vi "Pix Diff and Angle Info.vi"(6 "Split Image Info":T3={"height"=120.0, "width"=120.0, "deg/pix"=120.0}, 10 "Angle Mode":enum16{"Barrel View", "360 View"}(ring), 11 "located tags":T2(array[cluster])) -> ()   [LabVIEW 2025]
panel:
  out "angle":dbl
  in  "deg/pix":dbl=0.125
  out "X":dbl
  out "Array 2":cluster{"X":dbl, "Y":dbl}[](array[cluster])
  out "Array":T1(array[cluster])
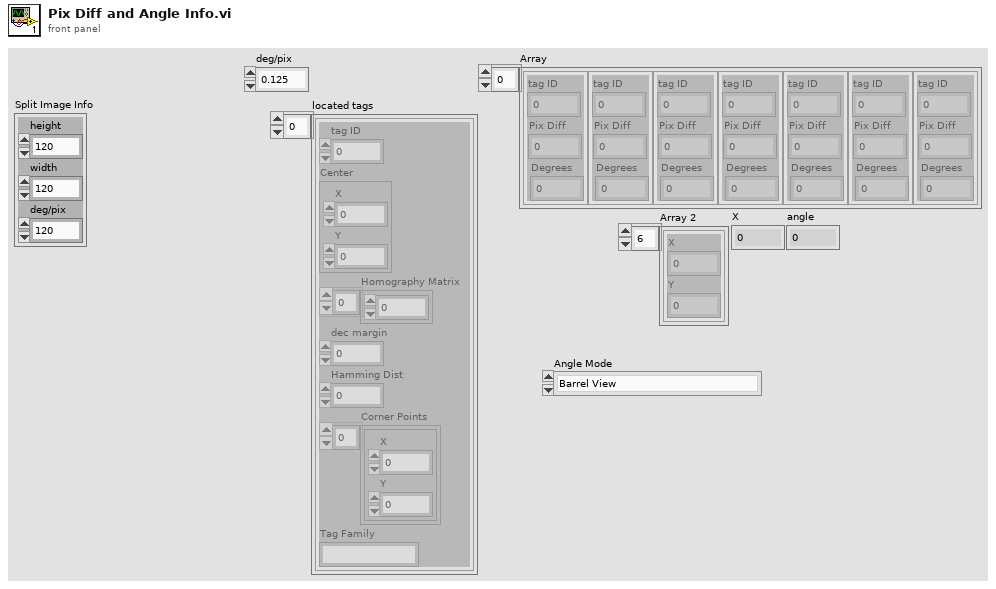
[diagram p1: front panel]
types:
  T1 = cluster{"tag ID":i32, "Pix Diff":dbl, "Degrees":dbl}[]
  T2 = cluster{"tag ID":i32, "Center":cluster{"X":dbl, "Y":dbl}, "Homography Matrix":dbl[], "dec margin":dbl, "Hamming Dist":i32, "Corner Points":cluster{"X":dbl, "Y":dbl}[], "Tag Family":string}[]
  T3 = cluster{"height":dbl, "width":dbl, "deg/pix":dbl}
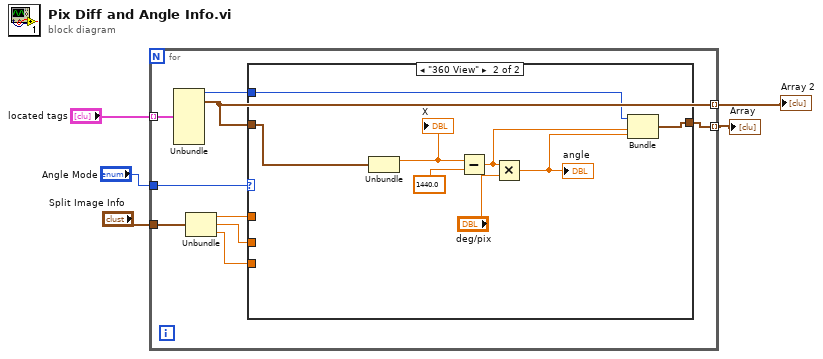
[diagram p0: block diagram]
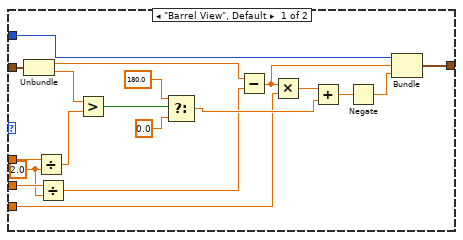
[diagram p2: hidden frame]
diagram:
  n1 = for {
    tunnel: "Split Image Info" -> [w14]
    tunnel: "located tags" -> [w10] mode=indexing
    tunnel: [w9] -> w3 mode=indexing
    tunnel: [w7] -> w2 mode=indexing
    tunnel: "Angle Mode" -> [w6]
    n2 = Unbundle(w10) -> ("tag ID"=w8:i32, "Center"=w7:cluster{"X":dbl, "Y":dbl})  [unwired: 5 out]
    n3 = Unbundle(w14) -> ("height"=w12:dbl, "width"=w13:dbl, "deg/pix"=w11:dbl)
    n4 = case shown="\"360 View\"" w6 {
      tunnel: w13 -> [w25 _]
      tunnel: w12 -> [w24 _]
      tunnel: w11 -> [w20 _]
      tunnel: [w19 w34] -> w9
      tunnel: w8 -> [w16 w37]
      tunnel: w7 -> [w15 w38]
      frame "Barrel View", Default {
        w23 = 2.0 ("y")
        n5 = Unbundle(w15) -> ("X"=w33:dbl, "Y"=w31:dbl)
        n6 = Divide(x=w24, y=w23) -> (x/y=w22:dbl)
        n7 = Divide(x=w25, y=w23) -> (x/y=w21:dbl)
        n8 = Greater?(x=w31, y=w22) -> (0:w32:bool)
        n9 = Select(t=180.0, s=w32, f=0.0) -> (s? t:f=w27:dbl)
        n10 = Subtract(x=w33, y=w21) -> (x-y=w18:dbl)
        n11 = Multiply(x=w18, y=w20) -> (x*y=w28:dbl)
        n12 = Add(x=w28, y=w27) -> (x+y=w26:dbl)
        n13 = Negate(x=w26) -> (-x=w17:dbl)
        n14 = Bundle("tag ID"=w16, w18, w17) -> (w19:cluster{"tag ID":i32, dbl, dbl})  [unwired: 1 in]
      }
      frame "360 View" {
        n15 = Unbundle(w38) -> ("X"=w41:dbl)  [unwired: 1 out]
        "X" <- w41
        n16 = Subtract(x=w41, y=1440.0) -> (x-y=w35:dbl)
        n17 = Multiply(x=w35, y="deg/pix") -> (x*y=w36:dbl)
        "angle" <- w36
        n18 = Bundle("tag ID"=w37, w35, w36) -> (w34:cluster{"tag ID":i32, dbl, dbl})  [unwired: 1 in]
      }
    }
  }
  "Array" <- w3
  "Array 2" <- w2
